vi "Add Subsystem to Tree.vi"(8 "error in (no error)":errorcluster, 9 "Subsystem I/O Attributes":T1[](array[typedef]), 10 "Subsystem":T4={"Name"="Control1", "Root URL"=""}, 11 "Tree Control":refnum<vi>) -> (0 "error out":errorcluster, 3 "dup Tree Control":refnum<vi>)   [LabVIEW 2024]
doc: "Adds a subsystem in the tree control."
uses:
  Controls/Server/Subsystem Configuration.ctl
  Controls/Server/Subsystem IO Attributes.ctl
  Controls/Server/Subsystem IO Logging Attributes.ctl
  Controls/Server/Subsystem IO Alarm Attributes.ctl
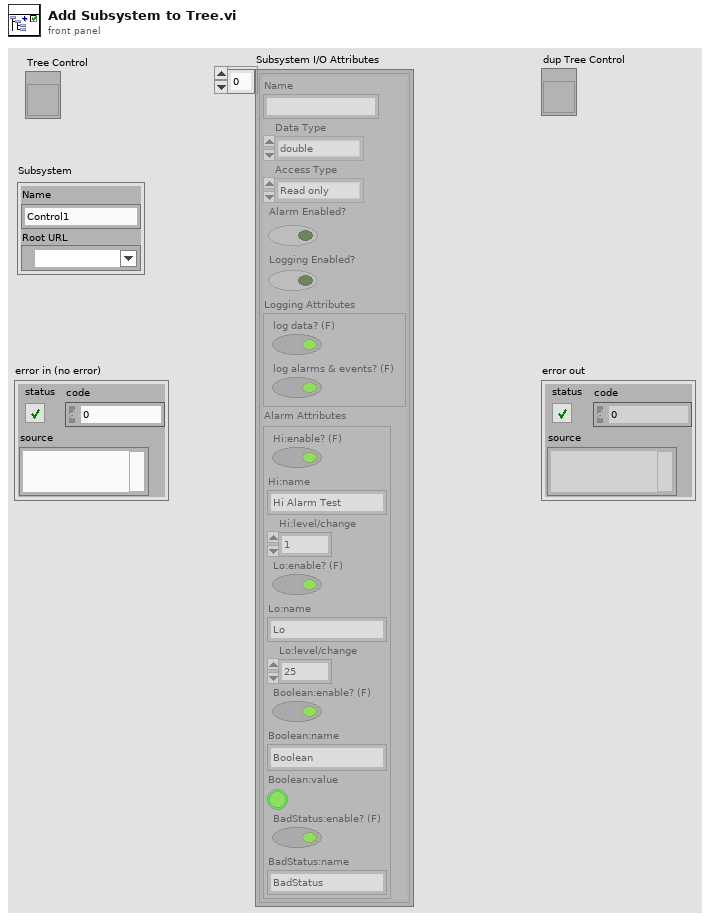
[diagram p1: front panel]
types:
  T1 = typedef "Subsystem IO Attributes.ctl" = cluster{"Name":string, "Data Type":enum32{"u32BitField", "bool", "double", "string", "int8", "uint8", "int16", "uint16", "int32", "uint32", "int64", "uint64", "single", "double waveform", "int16 waveform", "array of boolean", "array of int8", "array of uint8", "array of int16", "array of uint16", "array of int32", "array of uint32", "array of int64", "array of uint64", "array of single", "array of double", "array of double waveform", "array of int16 waveform", "array of string", "variant", "timestamp", "fixed point", "custom"}, "Access Type":enum32{"Read only", "Write only", "Read/write"}, "Alarm Enabled?":bool, "Logging Enabled?":bool, "Logging Attributes":T2, "Alarm Attributes":T3}
  T2 = typedef "Subsystem IO Logging Attributes.ctl" = cluster{"log data? (F)":bool, "log alarms & events? (F)":bool}
  T3 = typedef "Subsystem IO Alarm Attributes.ctl" = cluster{"Hi:enable? (F)":bool, "Hi:name":string, "Hi:level/change":dbl, "Lo:enable? (F)":bool, "Lo:name":string, "Lo:level/change":dbl, "Boolean:enable? (F)":bool, "Boolean:name":string, "Boolean:value":bool, "BadStatus:enable? (F)":bool, "BadStatus:name":string}
  T4 = typedef "Subsystem Configuration.ctl" = cluster{"Name":string, "Root URL":refnum<k21>}
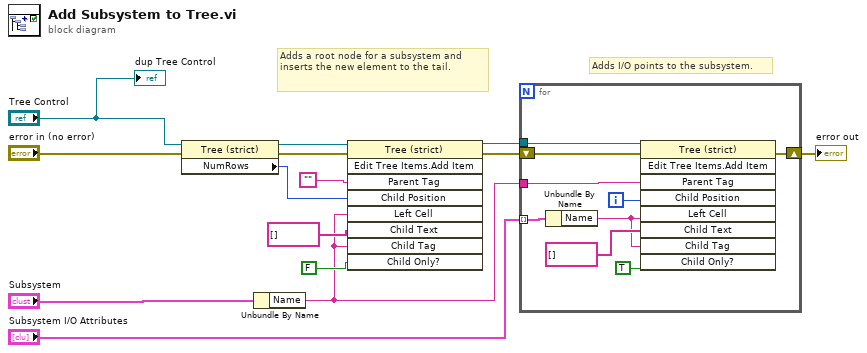
[diagram p0: block diagram]
diagram:
  # "Adds I/O points to the subsystem."
  # "Adds a root node for a subsystem and inserts the new element to the tail."
  n1 = property class="Tree (strict)"(reference="Tree Control", error in="error in (no error)") -> (reference out=w2:refnum<vi>, error out=w3:errorcluster, "NumRows"=w1:u32)
  n2 = Unbundle By Name("Subsystem") -> ("Name"=w4:string)
  n3 = invoke class="Tree (strict)" method="Edit Tree Items.Add Item"(reference=w2, error in=w3, "Parent Tag"="", "Child Position"=w1, "Left Cell"=w4, "Child Text"=string[] [], "Child Tag"=w4, "Child Only?"=FALSE) -> (reference out=w9:refnum<vi>, error out=w8:errorcluster)  [unwired: 1 in, 7 out]
  n4 = for {
    tunnel: "Subsystem I/O Attributes" -> [w18] mode=indexing
    shift-right: [w22] -> w13
    shift-left: w8 -> [w21]
    tunnel: w4 -> [w20]
    tunnel: w9 -> [w23]
    i -> [w19]
    n5 = Unbundle By Name(w18) -> ("Name"=w16:string)
    n6 = invoke class="Tree (strict)" method="Edit Tree Items.Add Item"(reference=w23, error in=w21, "Parent Tag"=w20, "Child Position"=w19, "Left Cell"=w16, "Child Text"=string[] [], "Child Tag"=w16, "Child Only?"=TRUE) -> (error out=w22:errorcluster)  [unwired: 1 in, 8 out]
  }
  "error out" <- w13
  "dup Tree Control" <- "Tree Control"
